vi "CSC_Set_Trans0toG.vi"(8 "error in (no error)":errorcluster, 10 "Real Matrix":T1, 11 "CableSerialChain in":refnum<class "CableSerialChain.lvclass">) -> (0 "error out":errorcluster, 3 "CableSerialChain out":refnum<class "CableSerialChain.lvclass">)   [LabVIEW 2015, in "CableSerialChain.lvclass"]
uses:
  CableSerialChain.lvclass
  <vilib>/Analysis/Matrix/Datatypes/RealMatrix.ctl
  CableSerialChain.lvclass/CableSerialChain.ctl
  <vilib>/Analysis/Matrix/NI_Matrix.lvlib
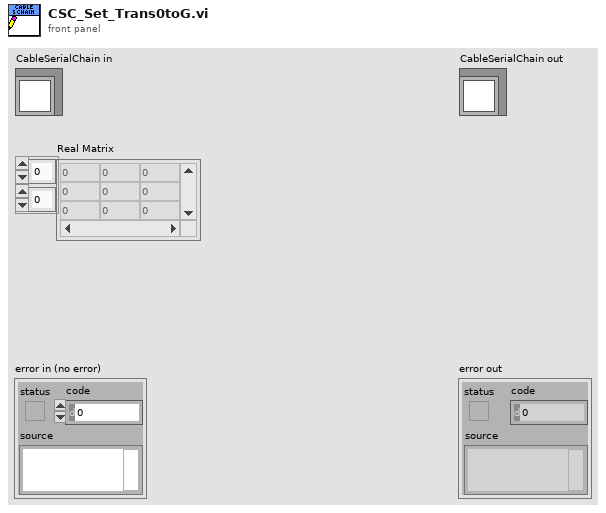
[diagram p1: front panel]
types:
  T1 = typedef "NI_Matrix.lvlib/RealMatrix.ctl" = dbl[][]
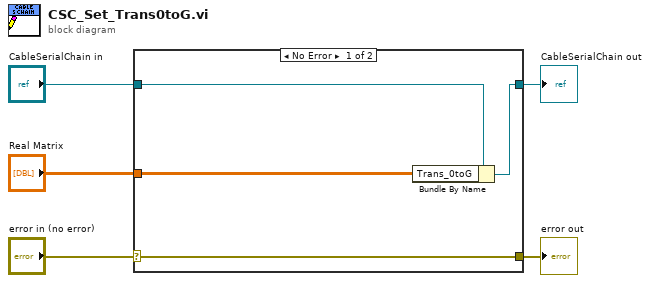
[diagram p0: block diagram]
diagram:
  n1 = case shown="No Error" "error in (no error)" {
    selector: "error in (no error)" -> [w9 w10]
    tunnel: [w9 w10] -> w4
    tunnel: [w7 w11] -> w2
    tunnel: "CableSerialChain in" -> [w8 w11]
    tunnel: "Real Matrix" -> [w6 _]
    frame No Error {
      n2 = Bundle By Name(cluster=w8, "Trans_0toG"=w6) -> (w7:refnum<class "CableSerialChain.lvclass">)
    }
    frame Error {
    }
  }
  "error out" <- w4
  "CableSerialChain out" <- w2
